vi "_010.vi"() -> ()   [LabVIEW 2024]
panel:
  out "Array 24":string[][][](array[string])
  out "Array 22":string[][][](array[string])
  in  "Array 23":string[][][](array[string])
  in  "Array 21":string[][][](array[string])
  out "Array 20":string[][](array[string])
  in  "Array 19":string[][](array[string])
  out "Array 18":string[](array[string])
  in  "Array 17":string[](array[string])
  out "Array 16":bool[][][][][](array[boolean])
  in  "Array 15":bool[][][][][](array[boolean])
  out "Array 14":bool[][][](array[boolean])
  in  "Array 13":bool[][][](array[boolean])
  out "Array 12":bool[][](array[boolean])
  in  "Array 11":bool[][](array[boolean])
  out "Array 10":bool[](array[boolean])
  in  "Array 9":bool[](array[boolean])
  out "Array 8":dbl[][][][](array[numeric])
  in  "Array 7":dbl[][][][](array[numeric])
  out "Array 6":dbl[][][](array[numeric])
  in  "Array 5":dbl[][][](array[numeric])
  out "Array 4":dbl[][](array[numeric])
  in  "Array 3":dbl[][](array[numeric])
  out "Array 2":dbl[](array[numeric])
  in  "Array":dbl[](array[numeric])
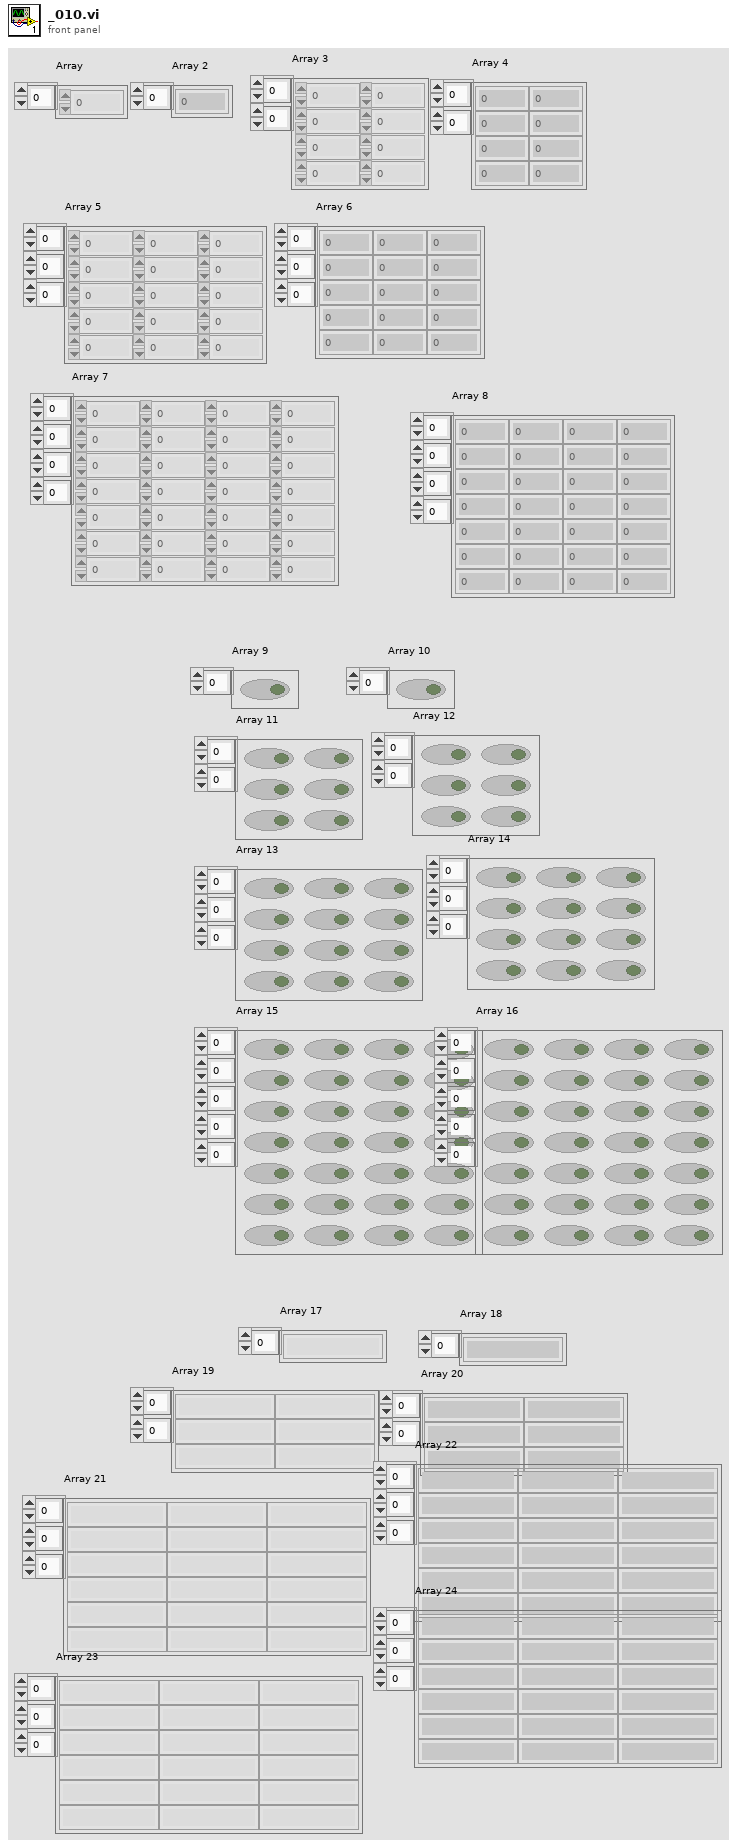
[diagram p1: front panel]
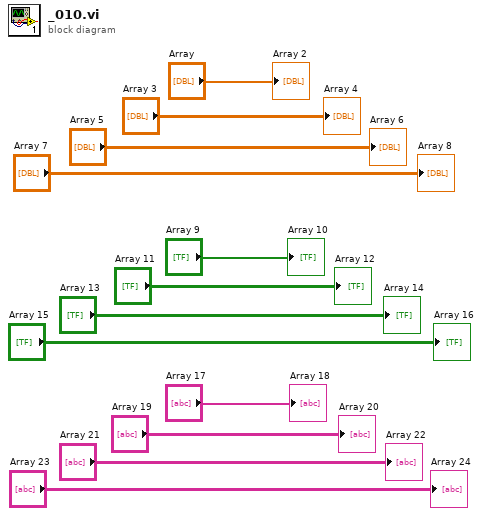
[diagram p0: block diagram]
diagram:
  "Array 2" <- "Array"
  "Array 4" <- "Array 3"
  "Array 6" <- "Array 5"
  "Array 8" <- "Array 7"
  "Array 10" <- "Array 9"
  "Array 12" <- "Array 11"
  "Array 14" <- "Array 13"
  "Array 16" <- "Array 15"
  "Array 18" <- "Array 17"
  "Array 20" <- "Array 19"
  "Array 22" <- "Array 21"
  "Array 24" <- "Array 23"
